vi "Read Control_delay_buffer.vi"(8 "error in (no error)":errorcluster, 11 "Model_Predictor in":refnum<class "Model_Predictor.lvclass">) -> (0 "error out":errorcluster, 2 "Control_delay_buffer":bool[](array[boolean]), 3 "Model_Predictor out":refnum<class "Model_Predictor.lvclass">)   [LabVIEW 2021, in "MBPOnOff_Controller.lvlib" / "Model_Predictor.lvclass"]
uses:
  Model_Predictor.lvclass
  Model_Predictor.lvclass/Model_Predictor.ctl
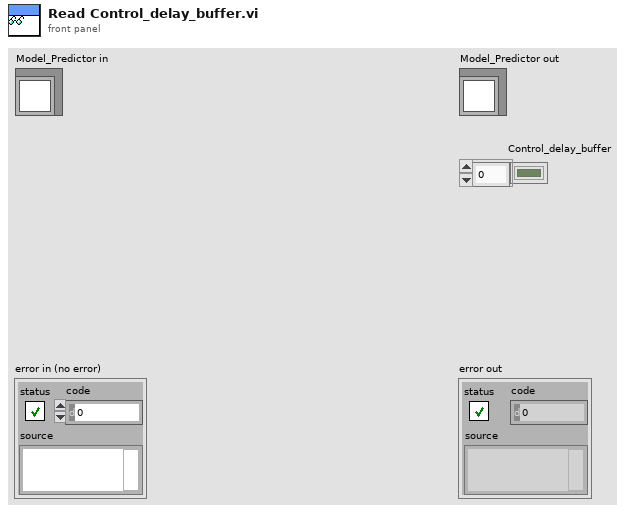
[diagram p1: front panel]
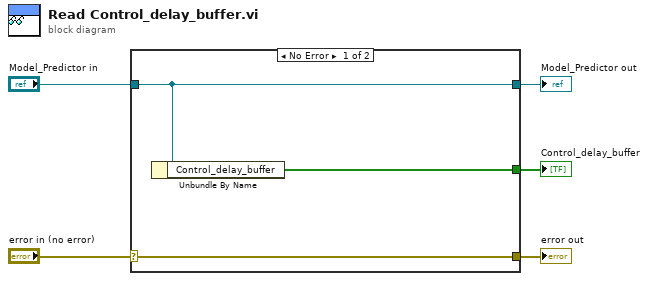
[diagram p0: block diagram]
diagram:
  n1 = case shown="No Error" "error in (no error)" {
    selector: "error in (no error)" -> [w8 w9]
    tunnel: [w8 w9] -> w4
    tunnel: [w7 w10] -> w2
    tunnel: "Model_Predictor in" -> [w7 w10]
    tunnel: [w6 _] -> w1
    frame No Error {
      n2 = Unbundle By Name(w7) -> ("Control_delay_buffer"=w6:bool[])
    }
    frame Error {
    }
  }
  "error out" <- w4
  "Model_Predictor out" <- w2
  "Control_delay_buffer" <- w1
